vi "WPI_RobotDriveMotors_3005.vi"(8 "error in":errorcluster, 9 "RightSpeed":dbl, 10 "LeftSpeed":dbl, 11 "RobotDriveDevRef":T1={"DevStatus"={"status"=FALSE, "code"=0, "source"=""}, "Motors[]"=[], "Square Inputs"=FALSE, "Max Output"=1.0, "Isochronous"=FALSE}) -> (0 "error out":errorcluster, 2 "Motor Values":dbl[](array[numeric]), 3 "RobotDriveDevRef":T1={"DevStatus"={"status"=FALSE, "code"=0, "source"=""}, "Motors[]"=[], "Square Inputs"=FALSE, "Max Output"=1.0, "Isochronous"=FALSE})   [LabVIEW 2013]
doc: "Determines the motor configuration and sends the speed values to the appropriate motors.\n\nThis software is licensed. Open the labview\\readme\\WPI Robotics Library Open Source License.txt file for more information."
uses:
  <vilib>/Rock Robotics/WPI/RobotDrive/WPI_RobotDriveDevRef.ctl
  <vilib>/Rock Robotics/WPI/MotorControl/WPI_MotorControlDeviceRef.ctl
  <vilib>/Rock Robotics/SystemInterfaces/Typedef/FPGA_TypedefDigitalModule.ctl
  <vilib>/Rock Robotics/SystemInterfaces/DIO/FPGA_DIOPWMChannel.ctl
  <vilib>/Rock Robotics/WPI/PWM/WPI_PWMDeadband.ctl
  <vilib>/Rock Robotics/WPI/CAN/Jaguar/SubVIs/WPI_CANJaguar_ControlMode.ctl
  <vilib>/Rock Robotics/WPI/PWM/WPI_PWMTransform_ConPane.ctl
  <vilib>/Rock Robotics/WPI/RobotDrive/WPI_RobotDriveSafetyCheck.vi
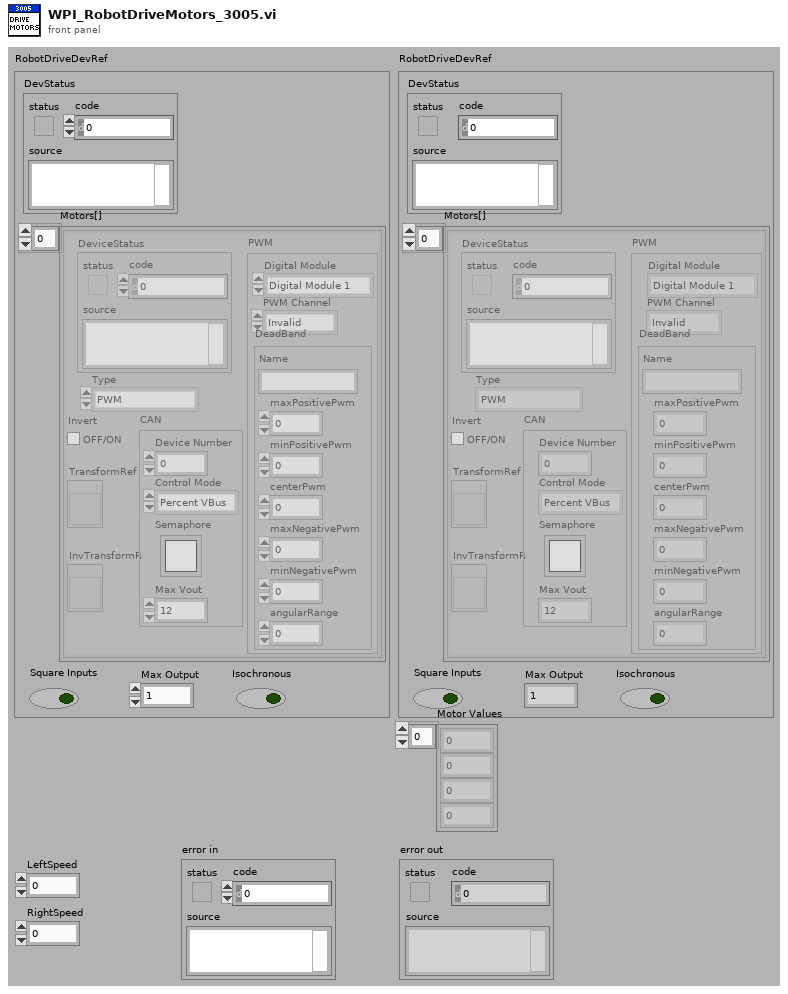
[diagram p1: front panel]
types:
  T1 = typedef "WPI_RobotDriveDevRef.ctl" = cluster{"DevStatus":errorcluster, "Motors[]":T2[], "Square Inputs":bool, "Max Output":dbl, "Isochronous":bool}
  T2 = typedef "WPI_MotorControlDeviceRef.ctl" = cluster{"DeviceStatus":errorcluster, "Type":enum16{"PWM", "CAN"}, "PWM":cluster{"Digital Module":T3, "PWM Channel":T4, "DeadBand":T5}, "CAN":cluster{"Device Number":u8, "Control Mode":T6, "Semaphore":T7, "Max Vout":dbl}, "Invert":bool, "TransformRef":T8, "InvTransformRef":T8}
  T3 = typedef "FPGA_TypedefDigitalModule.ctl" = enum16{"Digital Module 1", "Digital Module 2"}
  T4 = typedef "FPGA_DIOPWMChannel.ctl" = enum8{"PWM 1", "PWM 2", "PWM 3", "PWM 4", "PWM 5", "PWM 6", "PWM 7", "PWM 8", "PWM 9", "PWM 10", "Invalid"}
  T5 = typedef "WPI_PWMDeadband.ctl" = cluster{"Name":string, "maxPositivePwm":i32, "minPositivePwm":i32, "centerPwm":i32, "maxNegativePwm":i32, "minNegativePwm":i32, "angularRange":u16}
  T6 = typedef "WPI_CANJaguar_ControlMode.ctl" = enum8{"Percent VBus", "Current", "Speed", "Position", "Voltage"}
  T7 = typedef "Semaphore RefNum" = refnum<k1>
  T8 = typedef "WPI_PWMTransform_ConPane.ctl" = refnum<vi>
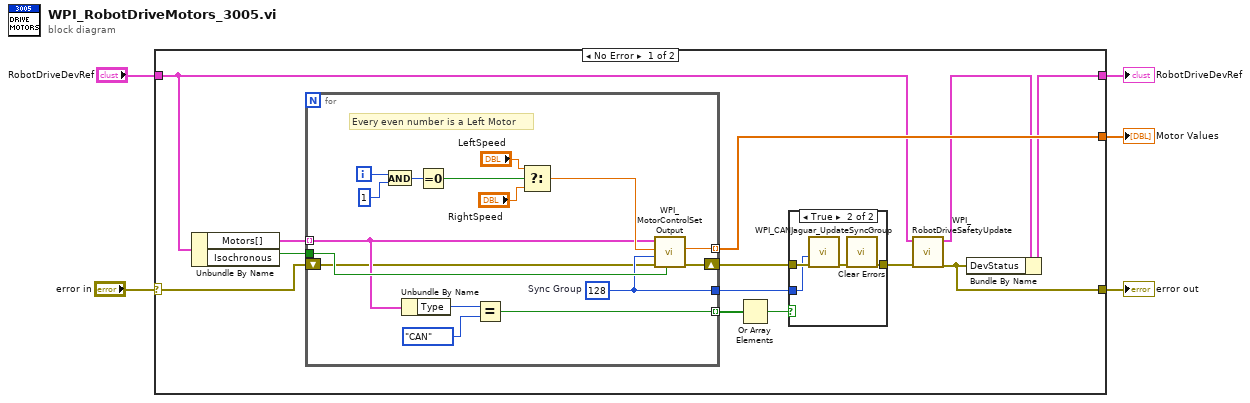
[diagram p0: block diagram]
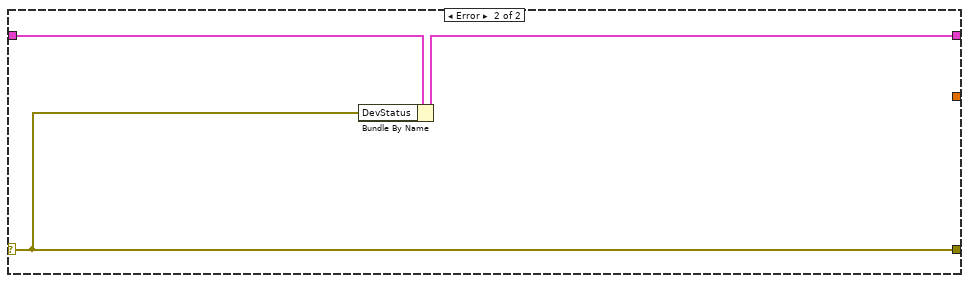
[diagram p3: hidden frame]
diagram:
  n1 = case shown="No Error" "error in" {
    selector: "error in" -> [w6 w40]
    tunnel: [w12 _] -> w5
    tunnel: "RobotDriveDevRef" -> [w10 w42]
    tunnel: [w8 w41] -> w3
    tunnel: [w7 w40] -> w2
    frame No Error {
      n2 = Unbundle By Name(w10) -> ("Motors[]"=w18:T2[], "Isochronous"=w17:bool)
      n3 = for {
        tunnel: [w39] -> w12 mode=indexing
        tunnel: w18 -> [w30] mode=indexing
        tunnel: w17 -> [w38]
        tunnel: [w27] -> w16 mode=indexing
        tunnel: [w26] -> w14
        shift-right: [w25] -> w13
        shift-left: w6 -> [w24]
        i -> [w37]
        w26 = u8 128  # Sync Group
        # "Every even number is a Left Motor"
        n4 = And(x=w37, y=1) -> (x .and. y?=w35:i32)
        n5 = Unbundle By Name(w30) -> ("Type"=w28:enum16{"PWM", "CAN"})
        n6 = Equal To 0?(x=w35) -> (x = 0?=w34:bool)
        n7 = Equal?(x=w28, y=enum16{"PWM", "CAN"}."CAN" ("Type")) -> (x = y?=w27:bool)
        n8 = Select(t="LeftSpeed", s=w34, f="RightSpeed") -> (s? t:f=w31:dbl)
        n9 = call <vilib>:"WPI_MotorControlSetOutput.vi"("Isochronous"=w38, "error in (no error)"=w24, "Sync Group"=w26, "Output"=w31, "MotorControlDevRef"=w30) -> ("error out"=w25:errorcluster, "Motor Output"=w39:dbl)  [unwired: 5 out]
      }
      n10 = Or Array Elements(Boolean array=w16) -> (logical OR=w15:bool)
      n11 = case shown="True" w15 {
        tunnel: w13 -> [w19 w22]
        tunnel: w14 -> [_ w21]
        tunnel: [w19 w20] -> w11
        frame False {
        }
        frame True {
          n12 = call <vilib>:"WPI_CANJaguar_UpdateSyncGroup.vi"("error in (no error)"=w22, "Sync Group"=w21) -> ("error out"=w23:errorcluster)  [unwired: 9 out]
          n13 = call <vilib>:"Clear Errors.vi"("error in (no error)"=w23) -> ("error out"=w20:errorcluster)  [unwired: 6 out]
        }
      }
      n14 = call <vilib>:"WPI_RobotDriveSafetyUpdate.vi"("error in (no error)"=w11, "RobotDriveDevRef"=w10) -> ("error out"=w7:errorcluster, "RobotDriveDevRef"=w9:T1)  [unwired: 8 out]
      n15 = Bundle By Name(cluster=w9, "DevStatus"=w7) -> (w8:T1)
    }
    frame Error {
      n16 = Bundle By Name(cluster=w42, "DevStatus"=w40) -> (w41:T1)
    }
  }
  "RobotDriveDevRef" <- w3
  "error out" <- w2
  "Motor Values" <- w5
